vi "写入原始数据数组.vi"(8 "error in (no error)":errorcluster caption="错误输入（无错误）", 11 "抽取参数输入":refnum<class "抽取参数.lvclass">) -> (0 "error out":errorcluster caption="错误输出", 3 "抽取参数输出":refnum<class "抽取参数.lvclass">)   [LabVIEW 2020, in "抽取参数.lvclass"]
uses:
  <vilib>/Utility/NIReport.llb/Report Type.ctl
  <vilib>/addons/_office/excel.llb/Excel Get Data ([str]).vi
  <vilib>/Utility/NIReport.llb/NI_report.lvclass
  <vilib>/addons/_office/NI_ReportGenerationToolkit.lvlib
  <vilib>/Utility/NIReport.llb/NI_ReportGenerationCore.lvlib
  <vilib>/Utility/NIReport.llb/Excel/NI_Excel.lvclass
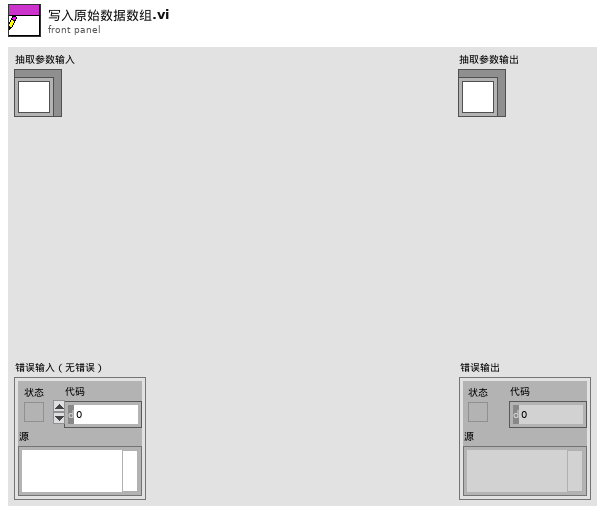
[diagram p1: front panel]
types:
  T1 = typedef "NI_ReportGenerationCore.lvlib/Report Type.ctl" = enum16{"HTML", "Word", "Excel"}
  T2 = enum16{"maximized", "minimized", "normal", "no change"}
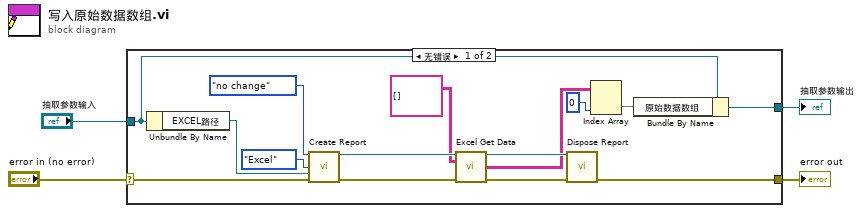
[diagram p0: block diagram]
diagram:
  n1 = case shown="无错误" "error in (no error)" {
    selector: "error in (no error)" -> [w6 w20]
    tunnel: [w5 w20] -> w3
    tunnel: [w19 w21] -> w1
    tunnel: "抽取参数输入" -> [w18 w21]
    frame No Error {
      n2 = Unbundle By Name(w18) -> ("EXCEL路径"=w15:path)
      n3 = call <vilib>:"Create Report.vi"("window state (normal)"=T2."no change", "report type"=Report_Type."Excel", "template (empty)"=w15, "error in (no error)"=w6) -> ("report out"=w14:refnum<class "NI_report.lvclass">, "error out"=w13:errorcluster)  [unwired: 10 in]
      n4 = call-poly <vilib>:"Excel Get Data.vi"("report in"=w14, "data type"=string[][] [], "error in (no error)"=w13) -> ("report out"=w11:refnum<class "NI_report.lvclass">, "data"=w9:string[][], "error out"=w10:errorcluster)  [unwired: 10 in]
      n5 = call-dynamic "Dispose Report.vi"("report in"=w11, "error in (no error)"=w10) -> ("error out"=w5:errorcluster)  [unwired: 13 in]
      n6 = Index Array(array=w9, index (col)=0 ("禁用的索引 (列)")) -> (element=w7:string[])  [unwired: 1 in]
      n7 = Bundle By Name(cluster=w18, "原始数据数组"=w7) -> (w19:refnum<class "抽取参数.lvclass">)
    }
    frame Error {
    }
  }
  "error out" <- w3
  "抽取参数输出" <- w1
